vi "BME_DG_Deactivate.vi"(8 "error in (no error)":errorcluster, 11 "DG_Number":i32) -> (0 "error out":errorcluster, 3 "return value":u32)   [LabVIEW 2009]
uses:
  BME DLL/DelayGenerator.dll
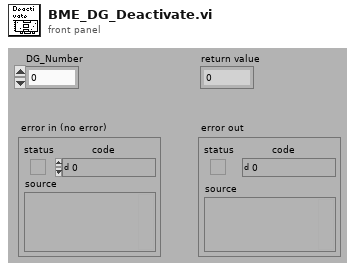
[diagram p1: front panel]
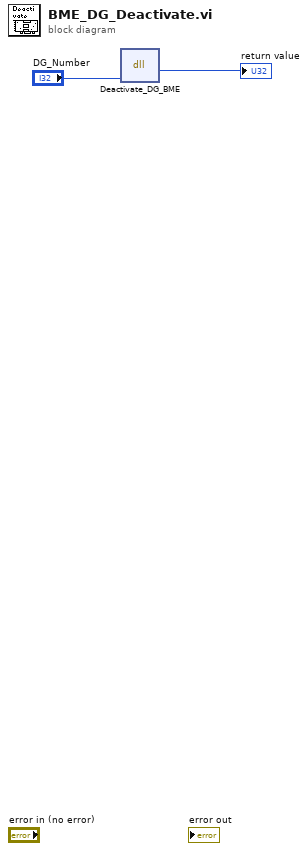
[diagram p0: block diagram]
diagram:
  n1 = dll-call lib="C:/Dokumente und Einstellungen/A2.5/Desktop/POLARIS BME DG/BME DLL/DelayGenerator.dll" fn="Deactivate_DG_BME"("DG_Number"="DG_Number") -> (→"return value":u32)  [unwired: 4 in, 2 out]
